vi "LineDetection-Hough.vi"() -> ()   [LabVIEW 2014]
doc: "This example shows how to use the Edge Tool in NI Vision. The Edge Tool finds edges (or sharp transitions in the pixels values) along a given line or ROI profile. The Edge Tool is a precursor function to many of the gauging and inspection tasks. For example, the location of the edges found along a line profile across an object can interpreted as the boundaries of the object whose dimensions have to be measured for a gauging application or the presence of a crack in the surface of an object for an inspection application."
uses:
  <vilib>/vision/Measure.llb/Edge Options.ctl
  <vilib>/vision/Measure.llb/Edge Polarity.ctl
  <vilib>/vision/Measure.llb/Straight Edge Options.ctl
  <vilib>/vision/Measure.llb/Straight Edge Process.ctl
  <vilib>/vision/NI_Vision_Development_Module.lvlib
panel:
  in  "Line Fit Options":T1={"Number of Lines"=1, "Type"=enum."First Edge Rake", "Min. Score"=10.0, "Max. Score"=1000.0, "Orientation"=0.0, "Angle Range"=45.0, "Angle Tolerance"=1.0, "Step Size"=7, "Min. SNR (db)"=0.0, "Min. Points (%)"=25.0, "Hough Iterations"=5} {"Min. Points (%)" min=0.0 max=100.0; "Min. SNR (db)" min=0.0; "Max. Score" min=0.0 max=1024.0; "Min. Score" min=0.0 max=1024.0 step=1.0}
  in  "Options":T5={"Search Direction"=0, "Edge Options"={"Edge Polarity"=0, "Kernel Size"=3, "Width"=3, "Minimum Edge Strength"=15.0, "Interpolation Type"=enum."Bilinear Fixed", "Data Processing Method"=enum."Average"}, "Show Search Area"=FALSE, "Show Search Lines"=FALSE, "Show Edges Found"=FALSE, "Show Result"=TRUE, "Search Area Color"=65280, "Search Lines Color"=255, "Edge Locations Color"=16776960, "Result Color"=16711680, "Overlay Group Name"=""} {"Edge Options"."Edge Polarity" items=["All Edges", "Rising Edges", "Falling Edges"]; "Edge Options"."Minimum Edge Strength" format="%.2f"; "Edge Options"."Width" step=2; "Edge Options"."Kernel Size" step=2; "Search Direction" items=["Left to Right", "Right to Left", "Top to Bottom", "Bottom to Top"]}
  out "Image":T6(plugin-control)
  in  "Stop":bool
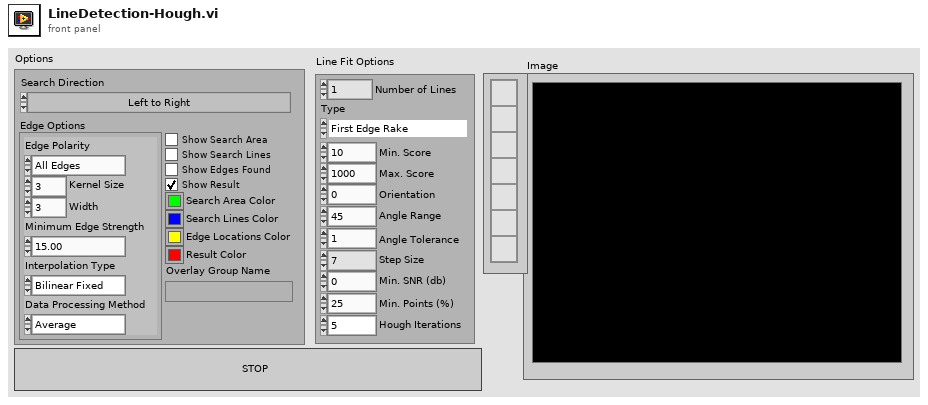
[diagram p1: front panel]
types:
  T1 = typedef "Straight Edge Options.ctl" = cluster{"Number of Lines":i32, "Type":T2, "Min. Score":dbl, "Max. Score":dbl, "Orientation":dbl, "Angle Range":dbl, "Angle Tolerance":dbl, "Step Size":u32, "Min. SNR (db)":dbl, "Min. Points (%)":dbl, "Hough Iterations":i32}
  T2 = typedef "Straight Edge Process.ctl" = enum32{"First Edge Rake", "Best Edge Rake", "Hough Edge Rake", "First Edge Projection", "Best Edge Projection"}
  T3 = typedef "Edge Options.ctl" = cluster{"Edge Polarity":T4, "Kernel Size":u32, "Width":u32, "Minimum Edge Strength":sgl, "Interpolation Type":enum32{"Zero Order", "Bilinear", "Quadratic", "Cubic", "Bilinear Fixed"}, "Data Processing Method":enum32{"Average", "Median"}}
  T4 = typedef "Edge Polarity.ctl" = u32
  T5 = cluster{"Search Direction":u32, "Edge Options":T3, "Show Search Area":bool, "Show Search Lines":bool, "Show Edges Found":bool, "Show Result":bool, "Search Area Color":u32, "Search Lines Color":u32, "Edge Locations Color":u32, "Result Color":u32, "Overlay Group Name":string}
  T6 = typedef "IMAQ Image.ctl" = refnum<image>
  T7 = typedef "IMAQ Rectangle" = cluster{"Left":i32, "Top":i32, "Right":i32, "Bottom":i32, "Rotation":dbl}
  T8 = typedef "ROI Descriptor" = cluster{"Global Rectangle":i32[], "Contours":cluster{"ID":enum32{"External", "Internal"}, "Type":u32, "Coordinates":i32[]}[]}
  T9 = cluster{"Options":cluster{"Search Direction":u32, "Edge Options":T3, "Show Search Area":bool, "Show Search Lines":bool, "Show Edges Found":bool, "Show Result":bool, "Search Area Color":u32, "Search Lines Color":u32, "Edge Locations Color":u32, "Result Color":u32, "Overlay Group Name":string}, "Line Fit Options":T1}
  T10 = cluster{"Global Rectangle":i32[], "Contours":cluster{"Contour Type":u32, "ROI Type":u32, "Points":i32[]}[]}
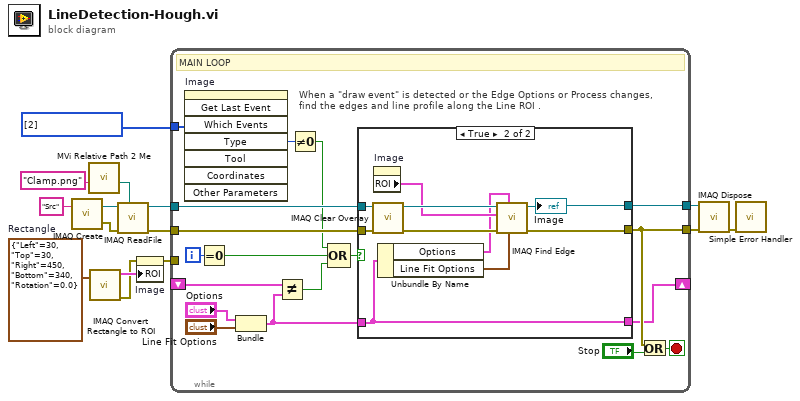
[diagram p0: block diagram]
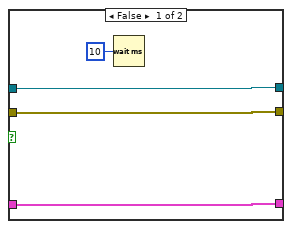
[diagram p2: hidden frame]
diagram:
  w1 = T7 {"Left"=30, "Top"=30, "Right"=450, "Bottom"=340, "Rotation"=0.0}  # Rectangle
  w7 = i32[] [2] items=["No  event", "Click event", "Draw event", "Move event", "Size event", "Scroll event", "Activate event", "Close event", "Double click event"] ("Events list (all)")
  n1 = call "IMAQ Create"("Image Name"="Src") -> ("New Image"=w14:T6, "error out"=w13:errorcluster)  [unwired: 4 in]
  n2 = call "MVi Relative Path 2 Me.vi"("Relative Path"="Clamp.png" ("name or relative path")) -> ("Appended Dir"=w5:path)  [unwired: 5 in, 1 out]
  n3 = call "IMAQ Convert Rectangle to ROI"("Rectangle"=w1) -> ("error out"=w3:errorcluster, "ROI Descriptor"=w4:T8)  [unwired: 8 in]
  n4 = call "IMAQ ReadFile"("File Path"=w5, "error in (no error)"=w13, "Image"=w14) -> ("error out"=w8:errorcluster, "Image Out"=w9:T6)  [unwired: 4 in, 3 out]
  n5 = property on="Image" class="ImageControl"(error in=w3, "ROI"=w4) -> (error out=w2:errorcluster)  [unwired: 1 in, 1 out]
  n6 = while "MAIN LOOP" {
    tunnel: w9 -> [w32]
    tunnel: w8 -> [w33]
    tunnel: [w28] -> w12
    tunnel: [w29] -> w11
    tunnel: w7 -> [w27]
    shift-right: [w22] -> _
    shift-left: _ -> [w19]
    tunnel: w2 -> [_]
    i -> [w25]
    stop <- w30 stop-if-true
    # "When a \"draw event\" is detected or the Edge Options or Process changes, find the edges and line profile along the Line ROI ."
    # "MAIN LOOP"
    n7 = invoke on="Image" class="ImageControl" method="Get Last Event"("Which Events"=w27) -> ("Type"=w26:i32)  [unwired: 7 in, 7 out]
    n8 = Equal To 0?(x=w25) -> (x = 0?=w21:bool)
    n9 = Bundle("Options"="Options", "Line Fit Options"="Line Fit Options") -> (w20:T9)  [unwired: 1 in]
    n10 = Not Equal?(x=w19, y=w20) -> (x != y?=w18:bool)
    n11 = Not Equal To 0?(x=w26) -> (x != 0?=w24:bool)
    n12 = Compound Arithmetic op=OR(w24, w21, w18) -> (w23:bool)
    n13 = case shown="True" w23 {
      tunnel: w33 -> [w36 w47]
      tunnel: w32 -> [w37 w46]
      tunnel: [w37 w38] -> w29
      tunnel: [w36 w39] -> w28
      tunnel: [w34 w45] -> w22
      tunnel: w20 -> [w34 w45]
      frame False {
        n14 = Wait (ms)(milliseconds to wait=u32 10) -> ()  [unwired: 1 out]
      }
      frame True {
        n15 = call "IMAQ Clear Overlay"("error in (no error)"=w47, "Image"=w46) -> ("error out"=w44:errorcluster, "Image Out"=w43:T6)  [unwired: 8 in]
        n16 = property on="Image" class="ImageControl"() -> ("ROI"=w41:T10)  [unwired: 2 in, 2 out]
        n17 = Unbundle By Name(w45) -> ("Options"=w40:T5, "Line Fit Options"=w42:T1)
        n18 = call "IMAQ Find Edge"("Line Fit Options"=w42, "Options"=w40, "error in (no error)"=w44, "ROI Descriptor"=w41, "Image"=w43) -> ("error out"=w39:errorcluster, "Image Out"=w38:T6)  [unwired: 3 in, 2 out]
        "Image" <- w38
      }
    }
    n19 = Or(x=w28, y="Stop") -> (x .or. y?=w30:bool)
  }
  n20 = call "IMAQ Dispose"("Image"=w11, "error in (no error)"=w12) -> ("error out"=w10:errorcluster)  [unwired: 4 in]
  n21 = call <vilib>:"Simple Error Handler.vi"("error in (no error)"=w10) -> ()  [unwired: 4 in, 5 out]
